vi "gyro-sweeper-V3.vi"() -> ()   [LabVIEW 2018]
uses:
  plot refs -- filter related.ctl
  cursor winow.ctl
  cursor window action.ctl
  KM_file -- read-write control.ctl
  agregator -- action.ctl
  circle corners.ctl
  lorentzian.ctl
  filename-action.ctl
  file -- read-write control.ctl
  publisher action.ctl
  show-win- control.ctl
  data source action.ctl
  cursor action.ctl
  2Dwindow.ctl
  sweper event.ctl
  filename-pattern.ctl
  freq scan type.ctl
  PLL data source.ctl
  peak -- parameters -- complex fit.ctl
  wavepacket.ctl
  filter method control.ctl
  parameters -- scan monitor control.ctl
panel:
  in  "start sweep! :r":bool
  in  "Tab :  Fit":enum32{"complex plane"}(tab)
  in  "fit!":bool=TRUE
  in  "plot staff!":enum16{"plot", "do not plot", "a"}(ring)
  in  "use fast fit!":bool
  out "# of points":dbl=953.475933538175
  out "win center (kHz)":dbl=3399.029286744401
  out "win width (kHz)":dbl=76.27809365793496
  in  "sweeper panel":enum32{"main", "parameters", "save scan"}(tab)
  in  "sweep! :r":bool
  in  "PLL data source":T1=enum."MFLI"
  out "Plot: circle sweep window":cluster{"all rows":dbl[], "all rows":dbl[]}[](graph)
  in  "win":T2={"cen (Hz)"=45005.0594236074, "win (Hz)"=127.23590686512762, "left (Hz)"=44941.44147017484, "right (Hz)"=45068.67737703997}
  in  "history length":i64=5
  out "fit is fine":bool=TRUE
  in  "gamma factor":dbl=1.6
  in  "scan type":T3
  in  "N":i64=250
  in  "Auto-update sweep window!":bool
  out "circle Q":dbl=4152.941585119393 format="%#11_11f"
  out "circle phase (rad)":dbl=0.3233468131446491 format="%#11_11f"
  out "circle gamma (Hz)":dbl=10.835608657224435 format="%#11_11f"
  out "circle frequency (Hz)":dbl=44999.649792667056 format="%#11_11f"
  in  "subtract bgnd!":bool
  in  "save data":enum32{"save/read"}(tab)
  in  "freqsweep name template":T4={"prefix"="RuCl3-rod", "group"="f"}
  in  "Save folder":path=path "/Users/Shared/Data"
  in  "freq sweep file name":string="f020_RuCl3-rod_042518.dat"
  in  "read from disk :l":bool
  in  "read file":path=path "/Users/arkady/Desktop/local_data/TaAs-quirk-Jan2018-losalamos/9w/f006_rucl3_012518.dat"
  in  "Tab :  Fit controls":T5(tab)
  in  "Plot: fragment - filter":cluster{dbl[], dbl[]}[](graph)=[{array[248 elements], array[248 elements]}, {array[248 elements], array[248 elements]}, {array[248 elements], array[248 elements]}, {array[248 elements], array[248 elements]}]
  out "Plot: phase around center":cluster{dbl[], dbl[]}[](graph)
  out "Plot: fragment":cluster{dbl[], dbl[]}[](graph)
  out "Plot: complex plane":cluster{dbl[], dbl[]}[](graph)=[{array[248 elements], array[248 elements]}, {[9.713674760263168e-05, 9.657708189915148e-05, 9.490691105118286e-05, 9.215257465070999e-05, 8.835751022812915e-05, 8.358156821644601e-05, 7.79000680741943e-05, 7.140261045258099e-05, 6.419166413969197e-05, 5.638095006649204e-05, 4.8093647859809984e-05, 3.9460453226039535e-05, 3.061751680177577e-05, 2.1704296976943485e-05, 1.2861360552679704e-05, 4.2281659189092685e-06, -4.059136287772788e-06, -1.186985036097273e-05, -1.9080796673861728e-05, -2.5578254295475043e-05, -3.125975443772674e-05, -3.6035696449409885e-05, -3.983076087199075e-05, -4.258509727246361e-05, -4.4255268120432224e-05, -4.481493382391242e-05, -4.4255268120432224e-05, -4.258509727246361e-05, -3.983076087199072e-05, -3.603569644940987e-05, -3.1259754437726735e-05, -2.5578254295475036e-05, -1.9080796673861714e-05, -1.1869850360972689e-05, -4.059136287772747e-06, 4.2281659189092685e-06, 1.2861360552679719e-05, 2.17042969769435e-05, 3.06175168017758e-05, 3.9460453226039576e-05, 4.809364785980996e-05, 5.638095006649204e-05, 6.419166413969198e-05, 7.1402610452581e-05, 7.790006807419431e-05, 8.358156821644603e-05, 8.835751022812915e-05, 9.215257465071001e-05, 9.490691105118286e-05, 9.657708189915148e-05], [-6.0789908179408565e-05, -5.1894276557869184e-05, -4.3138934360994235e-05, -3.466195856541634e-05, -2.6597036143331644e-05, -1.907135573908757e-05, -1.2203601828282588e-05, -6.102082992687433e-06, -8.630238292101184e-07, 3.430952569479092e-06, 6.712127630475673e-06, 8.928755262988767e-06, 1.0045877925104457e-05, 1.0045877925104457e-05, 8.928755262988753e-06, 6.712127630475673e-06, 3.4309525694790785e-06, -8.630238292101251e-07, -6.102082992687433e-06, -1.2203601828282601e-05, -1.9071355739087562e-05, -2.659703614333165e-05, -3.466195856541635e-05, -4.3138934360994235e-05, -5.18942765578692e-05, -6.0789908179408586e-05, -6.968553980094795e-05, -7.844088199782291e-05, -8.691785779340081e-05, -9.498278021548549e-05, -0.00010250846061972958, -0.00010937621453053454, -0.00011547773336612971, -0.00012071679252960703, -0.00012501076892829625, -0.00012829194398929282, -0.0001305085716218059, -0.0001316256942839216, -0.0001316256942839216, -0.00013050857162180587, -0.00012829194398929282, -0.00012501076892829622, -0.000120716792529607, -0.00011547773336612968, -0.00010937621453053451, -0.00010250846061972952, -9.498278021548549e-05, -8.691785779340079e-05, -7.844088199782288e-05, -6.968553980094791e-05]}, {[3.6089221403832686e-06, 5.864120615280904e-06, 8.11931909017854e-06, 1.0374517565076178e-05, 1.2629716039973813e-05, 1.4884914514871449e-05, 1.7140112989769086e-05, 1.939531146466672e-05, 2.1650509939564358e-05, 2.3905708414461995e-05, 2.616090688935963e-05, 2.8416105364257267e-05, 3.0671303839154904e-05, 3.292650231405254e-05, 3.518170078895017e-05, 3.743689926384781e-05, 3.969209773874545e-05, 4.194729621364308e-05, 4.420249468854072e-05, 4.6457693163438356e-05], [6.507773421354634e-06, -2.219947387216864e-07, -6.951762898798007e-06, -1.3681531058874325e-05, -2.0411299218950647e-05, -2.714106737902697e-05, -3.3870835539103284e-05, -4.0600603699179606e-05, -4.733037185925593e-05, -5.406014001933225e-05, -6.078990817940857e-05, -6.75196763394849e-05, -7.424944449956121e-05, -8.097921265963752e-05, -8.770898081971384e-05, -9.443874897979018e-05, -0.0001011685171398665, -0.00010789828529994281, -0.00011462805346001913, -0.00012135782162009547]}, {[9.345858849012286e-05, 8.672882033004654e-05, 7.999905216997021e-05, 7.32692840098939e-05, 6.653951584981757e-05, 5.980974768974125e-05, 5.307997952966494e-05, 4.6350211369588616e-05, 3.9620443209512294e-05, 3.289067504943597e-05, 2.616090688935965e-05, 1.9431138729283335e-05, 1.270137056920702e-05, 5.971602409130691e-06, -7.581657509456245e-07, -7.487933911021953e-06, -1.4217702071098268e-05, -2.0947470231174584e-05, -2.7677238391250912e-05, -3.440700655132724e-05], [-3.82379234304322e-05, -4.049312190532983e-05, -4.274832038022747e-05, -4.5003518855125107e-05, -4.725871733002275e-05, -4.951391580492038e-05, -5.1769114279818016e-05, -5.402431275471565e-05, -5.627951122961329e-05, -5.853470970451093e-05, -6.0789908179408565e-05, -6.30451066543062e-05, -6.530030512920383e-05, -6.755550360410147e-05, -6.981070207899912e-05, -7.206590055389675e-05, -7.432109902879438e-05, -7.657629750369202e-05, -7.883149597858965e-05, -8.10866944534873e-05]}, {[0.013424540165209643, 0.01681254433898315, 0.02019004611768062, 0.02355493467263274, 0.026905107058024576, 0.030238469525168014, 0.03355293883102678, 0.03684644354017529, 0.04011692531937857, 0.0433623402239834, 0.04658065997531719, 0.049769873228296214, 0.05292798682845071, 0.056053027057581604, 0.0591430408672702, 0.06219609709946967, 0.06521028769341622, 0.0681837288781047, 0.07111456234958441, 0.07400095643233846], [-0.13571760315957762, -0.13533981585140645, -0.1348774553139278, -0.13433081050742715, -0.13370022306711446, -0.13298608708961343, -0.1321888488866639, -0.13130900670619147, -0.13034711042091882, -0.12930376118471318, -0.12817961105688472, -0.1269753625946706, -0.1256917684141598, -0.12432963071993232, -0.12288980080370752, -0.1213731785123146, -0.11978071168531748, -0.11811339556264598, -0.11637227216260333, -0.1145584296306385]}, {[0.01490037751444529, 0.01866106214733388, 0.022410089121688074, 0.02614511541768493, 0.029863806765469864, 0.033563839103999085, 0.037242900033502314, 0.040898690260657164, 0.0445289250355728, 0.048131335579684166, 0.051703670503664666, 0.05524369721447139, 0.05874920331064287, 0.06221799796497817, 0.06564791329373253, 0.06903680571147393, 0.0723825572707546, 0.07568307698575881, 0.07893630213910129, 0.08214019957095828], [-0.15064482340041957, -0.15022547948834955, -0.14971225929174828, -0.14910548355653253, -0.14840553149778546, -0.1476128405627593, -0.14672790615748532, -0.14575128133716095, -0.1446835764605083, -0.14352545880832002, -0.14227765216643043, -0.14094093637337277, -0.13951614683300578, -0.13800417399241327, -0.13640596278540376, -0.13472251204195762, -0.1329548738639908, -0.13110415296782546, -0.1291715059937781, -0.12715814078329715]}, {array[248 elements], array[248 elements]}]
  in  "scale gauge: Plot: complex plane":dbl(slide)=0.00275 min=0.0 max=0.3 step=1e-06 scale=1e-05..0.5 scale format="%#_2g"
  out "lorentzian":T6={"A (VHz)"=0.0007690664340865132, "f (Hz)"=44999.649792667056, "G (Hz)"=10.835608657224435, "phi(rad)"=0.3233468131446491, "Q"=4152.941585119393, "Norm  Ampl"=nan, "bg (V)"=3.608922140383272e-06+6.507773421354641e-06i, "4corners"={"z (-pi/2)"=9.345858849012286e-05-3.8237923430432204e-05i, "z(inf)"=3.608922140383272e-06+6.507773421354641e-06i, "z (pi/2)"=-4.113677471140356e-05-8.334189292838493e-05i, "z center"=2.616090688935963e-05-6.0789908179408565e-05i, "z(0)"=4.871289163833599e-05-0.00012808758978017178i, "radius"=7.097584071327205e-05}} {"bg (V)" format="%#9_9f"; "Q" format="%#9_9f"; "phi(rad)" format="%#9_9f"; "G (Hz)" format="%#9_9f"; "f (Hz)" format="%#9_9f"}
  out "Plot: phase":cluster{"omega out":dbl[], dbl[]}(graph)
  out "Plot: win omega":T8(graph)
  out "Plot: dz/domega":cluster{"omega out":dbl[], dbl[]}(graph)
  in  "Plot: complex plane - filter":cluster{dbl[], dbl[]}[](graph)=[{array[248 elements], array[248 elements]}, {array[248 elements], array[248 elements]}, {[0.0001012150693760883, 0.00010107110703326549, 0.00010063978815839399, 9.992281497002211e-05, 9.892301703377042e-05, 9.764434009532913e-05, 9.609183050840228e-05, 9.427161531905536e-05, 9.219087808506348e-05, 8.985783052569077e-05, 8.728168011378607e-05, 8.447259373809396e-05, 8.144165757918983e-05, 7.820083335738984e-05, 7.476291112530571e-05, 7.114145879135017e-05, 6.73507685734012e-05, 6.340580059394736e-05, 5.932212383931916e-05, 5.511585471601265e-05, 5.080359344659598e-05, 4.6402358556214715e-05, 4.192951970824826e-05, 3.740272915418386e-05, 3.283985206824449e-05, 2.8258896041708113e-05, 2.367794001517175e-05, 1.9115062929232377e-05, 1.458827237516796e-05, 1.0115433527201521e-05, 5.7141986368202625e-06, 1.4019373674035856e-06, -2.8043317559029232e-06, -6.8880085105311325e-06, -1.0832976489984969e-05, -1.4623666707933929e-05, -1.8245119041889463e-05, -2.1683041273973607e-05, -2.4923865495773593e-05, -2.795480165467773e-05, -3.0763888030369817e-05, -3.334003844227453e-05, -3.5673086001647226e-05, -3.775382323563912e-05, -3.9574038424986043e-05, -4.112654801191287e-05, -4.240522495035418e-05, -4.340502288660586e-05, -4.412199607497775e-05, -4.455331494984924e-05, -4.469727729267206e-05, -4.455331494984924e-05, -4.412199607497775e-05, -4.340502288660585e-05, -4.240522495035418e-05, -4.112654801191287e-05, -3.957403842498603e-05, -3.7753823235639105e-05, -3.567308600164721e-05, -3.334003844227452e-05, -3.07638880303698e-05, -2.7954801654677702e-05, -2.4923865495773586e-05, -2.1683041273973594e-05, -1.824511904188945e-05, -1.4623666707933943e-05, -1.0832976489984928e-05, -6.888008510531119e-06, -2.8043317559028826e-06, 1.4019373674035991e-06, 5.7141986368202625e-06, 1.0115433527201551e-05, 1.4588272375167974e-05, 1.9115062929232425e-05, 2.3677940015171765e-05, 2.825889604170811e-05, 3.283985206824452e-05, 3.7402729154183855e-05, 4.1929519708248304e-05, 4.640235855621473e-05, 5.080359344659596e-05, 5.511585471601268e-05, 5.9322123839319156e-05, 6.34058005939474e-05, 6.735076857340121e-05, 7.114145879135022e-05, 7.476291112530574e-05, 7.820083335738984e-05, 8.144165757918985e-05, 8.447259373809397e-05, 8.72816801137861e-05, 8.98578305256908e-05, 9.219087808506348e-05, 9.427161531905536e-05, 9.609183050840228e-05, 9.764434009532913e-05, 9.892301703377042e-05, 9.992281497002211e-05, 0.00010063978815839399, 0.00010107110703326549], [-6.548300655616225e-05, -6.090205052962588e-05, -5.6339173443686514e-05, -5.1812382889622106e-05, -4.7339544041655654e-05, -4.2938309151274406e-05, -3.862604788185772e-05, -3.4419778758551206e-05, -3.0336102003923004e-05, -2.639113402446918e-05, -2.2600443806520194e-05, -1.8978991472564666e-05, -1.5541069240480522e-05, -1.2300245018680544e-05, -9.269308859776414e-06, -6.460222484084306e-06, -3.8840720721795965e-06, -1.5510245128068904e-06, 5.297127211849887e-07, 2.3499279105319138e-06, 3.902437497458743e-06, 5.18111443590005e-06, 6.1809123721517315e-06, 6.897885560523619e-06, 7.32920443539511e-06, 7.4731667782179325e-06, 7.32920443539511e-06, 6.897885560523619e-06, 6.180912372151718e-06, 5.18111443590005e-06, 3.902437497458743e-06, 2.3499279105319002e-06, 5.297127211849751e-07, -1.5510245128069175e-06, -3.88407207217961e-06, -6.460222484084306e-06, -9.269308859776414e-06, -1.230024501868055e-05, -1.5541069240480543e-05, -1.897899147256468e-05, -2.2600443806520187e-05, -2.639113402446918e-05, -3.0336102003923017e-05, -3.441977875855123e-05, -3.862604788185773e-05, -4.293830915127442e-05, -4.7339544041655654e-05, -5.1812382889622106e-05, -5.633917344368653e-05, -6.09020505296259e-05, -6.548300655616228e-05, -7.006396258269862e-05, -7.462683966863799e-05, -7.915363022270241e-05, -8.362646907066887e-05, -8.802770396105013e-05, -9.233996523046681e-05, -9.654623435377329e-05, -0.00010062991110840151, -0.00010457487908785534, -0.00010836556930580432, -0.00011198702163975986, -0.00011542494387184398, -0.00011866576809364396, -0.0001216967042525481, -0.0001245057906282402, -0.00012708194104014492, -0.0001294149885995176, -0.0001314957258335095, -0.00013331594102285643, -0.00013486845060978325, -0.00013614712754822457, -0.00013714692548447624, -0.0001378638986728481, -0.00013829521754771962, -0.00013843917989054242, -0.00013829521754771962, -0.0001378638986728481, -0.0001371469254844762, -0.00013614712754822457, -0.00013486845060978325, -0.0001333159410228564, -0.00013149572583350948, -0.00012941498859951757, -0.0001270819410401449, -0.00012450579062824017, -0.00012169670425254808, -0.00011866576809364396, -0.00011542494387184395, -0.00011198702163975983, -0.00010836556930580426, -0.0001045748790878553, -0.00010062991110840151, -9.654623435377327e-05, -9.233996523046677e-05, -8.802770396105006e-05, -8.362646907066882e-05, -7.91536302227024e-05, -7.462683966863795e-05, -7.006396258269862e-05]}, {[1.899482972370191e-05, 2.042190570156003e-05, 2.536299500300297e-06], [2.1388142418474606e-05, -4.9882036450666976e-05, 1.9102624564056266e-05]}, {[1.6088173004516162e-05, 1.5315829542932655e-05, 1.454348608134915e-05, 1.3771142619765645e-05, 1.299879915818214e-05, 1.2226455696598635e-05, 1.1454112235015128e-05, 1.0681768773431623e-05, 9.909425311848118e-06, 9.13708185026461e-06, 8.364738388681106e-06, 7.5923949270976005e-06, 6.820051465514094e-06, 6.0477080039305886e-06, 5.2753645423470834e-06, 4.503021080763577e-06, 3.7306776191800715e-06, 2.9583341575965664e-06, 2.1859906960130596e-06, 1.4136472344295545e-06], [2.141229803815197e-05, 2.129057954122817e-05, 2.116886104430437e-05, 2.104714254738057e-05, 2.0925424050456767e-05, 2.0803705553532967e-05, 2.0681987056609167e-05, 2.0560268559685368e-05, 2.0438550062761568e-05, 2.0316831565837768e-05, 2.0195113068913965e-05, 2.0073394571990165e-05, 1.9951676075066366e-05, 1.9829957578142566e-05, 1.9708239081218766e-05, 1.9586520584294966e-05, 1.9464802087371166e-05, 1.9343083590447363e-05, 1.9221365093523564e-05, 1.9099646596599764e-05]}, {[2.0421905701560028e-05, 2.1435595251954573e-05, 2.2449284802349118e-05, 2.3462974352743663e-05, 2.447666390313821e-05, 2.5490353453532754e-05, 2.6504043003927302e-05, 2.7517732554321847e-05, 2.8531422104716392e-05, 2.9545111655110937e-05, 3.055880120550548e-05, 3.157249075590003e-05, 3.2586180306294576e-05, 3.359986985668912e-05, 3.4613559407083666e-05, 3.562724895747821e-05, 3.664093850787276e-05, 3.76546280582673e-05, 3.866831760866185e-05, 3.968200715905639e-05], [-4.9882036450666976e-05, -4.9882036450666976e-05, -4.9882036450666976e-05, -4.9882036450666976e-05, -4.9882036450666976e-05, -4.9882036450666976e-05, -4.9882036450666976e-05, -4.9882036450666976e-05, -4.9882036450666976e-05, -4.9882036450666976e-05, -4.9882036450666976e-05, -4.9882036450666976e-05, -4.9882036450666976e-05, -4.9882036450666976e-05, -4.9882036450666976e-05, -4.9882036450666976e-05, -4.9882036450666976e-05, -4.9882036450666976e-05, -4.9882036450666976e-05, -4.9882036450666976e-05]}]
  in  "scale gauge: Plot: complex plane - filter":dbl(slide)=0.000254 min=0.0 max=0.3 step=1e-06 scale=1e-05..0.5 scale format="%#_5g"
  in  "scan monitor control":T9={"gamma acc. frac. - min "=0.3, "gamma acc frac.. - max"=3.0, "peak acc. fraction (af)"=5.0, "min peak acc. window (kHz)"=0.5, "use"=enum."fraction", "abs gamma min(kHz)"=0.005, "abs gamma max(kHz)"=5.0, "# points"=5, "gamma-factor (fa)"=3.0, "interpolate"=enum."line", "init"=TRUE, "Unique strike parameters"=TRUE, "max peak acc. window (kHz)"=10.0, "spacing factor"=1.5, "iterate #"=1, "overwrite ctl?"=FALSE, "write _m files?"=FALSE, "max slope (kHz/sweep)"=0.5, "funnel state"=enum."funnel open"}
  in  "parameters: complex fit":T10={"main VI path"=path "", "scale factor"=3.0, "# of grid points"=200, "parameters: wavepacket"={"R"=0.5, "wave number"=22.0, "delta k"=7.0, "radii vector"=[], "radial section"=[], "wave vector"=22.0, "wavepacket is"=TRUE}, "span"=0.27789, "interference ?"=enum."cp z center", "filter method"=enum."three"} {"span" min=0.0 max=0.5 step=1e-05 scale=0.0001..0.5 scale format="%#_5f"; "parameters: wavepacket"."delta k" format="%#_3f"; "parameters: wavepacket"."wave number" format="%#_3f"; "parameters: wavepacket"."R" format="%#_3f"}
  in  "cursor bracket: fit boundaries":T13={"left"=44877.82351674229, "right "=45005.05942360742, "center"=44941.441470174854, "window"=127.23590686512762, "cursors"=[3, 4, 5], "relative"=0, "absolute"=0, "fixed vertical offset"=0.0, "vertical offset"=0.0, "skew"=0.0, "default window frac"=0.1, "kind"=enum."symmetric", "skew.left"=0.5, "skew.right"=0.5, "Plot ref"=refnum, "wing order"=enum."forw"}
  in  "cursor bracket: circle window":T13={"left"=44941.44147017484, "right "=45068.67737703997, "center"=45005.0594236074, "window"=127.23590686512762, "cursors"=[0, 1, 2], "relative"=0, "absolute"=0, "fixed vertical offset"=0.0, "vertical offset"=0.0, "skew"=0.0, "default window frac"=0.1, "kind"=enum."symmetric", "skew.left"=0.5, "skew.right"=0.5, "Plot ref"=refnum, "wing order"=enum."forw"}
  # "three strikes"
  # "search window"
  # "linear extrapolation"
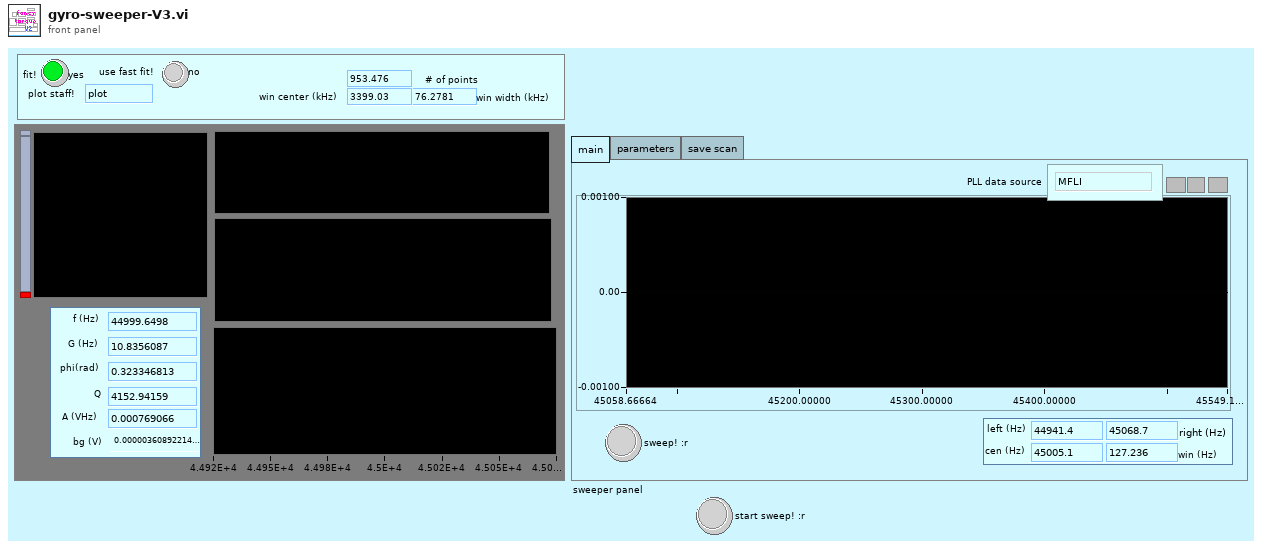
[diagram p1: front panel]
types:
  T1 = typedef "PLL data source.ctl" = enum16{"meta", "MFLI", "SRS865A"}
  T2 = typedef "show-win- control.ctl" = cluster{"cen (Hz)":dbl, "win (Hz)":dbl, "left (Hz)":dbl, "right (Hz)":dbl}
  T3 = typedef "freq scan type.ctl" = enum16{"linear", "arctan"}
  T4 = typedef "filename-pattern.ctl" = cluster{"prefix":string, "group":string}
  T5 = enum32{"complex plane", "complex plane 3", "complex plane 4"}
  T6 = typedef "lorentzian.ctl" = cluster{"A (VHz)":dbl, "f (Hz)":dbl, "G (Hz)":dbl, "phi(rad)":dbl, "Q":dbl, "Norm  Ampl":dbl, "bg (V)":cdb, "4corners":T7}
  T7 = typedef "circle corners.ctl" = cluster{"z (-pi/2)":cdb, "z(inf)":cdb, "z (pi/2)":cdb, "z center":cdb, "z(0)":cdb, "radius":dbl}
  T8 = cluster{"omega out":dbl[], "win omega out":dbl[]}
  T9 = typedef "parameters -- scan monitor control.ctl" = cluster{"gamma acc. frac. - min ":dbl, "gamma acc frac.. - max":dbl, "peak acc. fraction (af)":dbl, "min peak acc. window (kHz)":dbl, "use":enum16{"window", "fraction"}, "abs gamma min(kHz)":dbl, "abs gamma max(kHz)":dbl, "# points":i32, "gamma-factor (fa)":dbl, "interpolate":enum16{"line", "last"}, "init":bool, "Unique strike parameters":bool, "max peak acc. window (kHz)":dbl, "spacing factor":dbl, "iterate #":i32, "overwrite ctl?":bool, "write _m files?":bool, "max slope (kHz/sweep)":dbl, "funnel state":enum16{"funnel open", "funnel closed"}}
  T10 = typedef "peak -- parameters -- complex fit.ctl" = cluster{"main VI path":path, "scale factor":dbl, "# of grid points":i32, "parameters: wavepacket":T11, "span":dbl, "interference ?":enum16{"cp z center", "pm zcenter", "fancy"}, "filter method":T12}
  T11 = typedef "wavepacket.ctl" = cluster{"R":dbl, "wave number":dbl, "delta k":dbl, "radii vector":dbl[], "radial section":cdb[], "wave vector":dbl, "wavepacket is":bool}
  T12 = typedef "filter method control.ctl" = enum16{"four", "five", "one", "two", "three", "zero", "minus one", "minus two"}
  T13 = typedef "cursor winow.ctl" = cluster{"left":dbl, "right ":dbl, "center":dbl, "window":dbl, "cursors":i32[], "relative":i32, "absolute":i32, "fixed vertical offset":dbl, "vertical offset":dbl, "skew":dbl, "default window frac":dbl, "kind":enum16{"symmetric", "skewed", "fancy"}, "skew.left":dbl, "skew.right":dbl, "Plot ref":refnum<vi>, "wing order":enum16{"forw", "back"}}
  T14 = typedef "sweper event.ctl" = enum16{"sweep!", "stop"}
  T15 = typedef "publisher action.ctl" = enum16{"set", "get", "init", "check"}
  T16 = typedef "data source action.ctl" = enum16{"set", "get", "init", "set-and-get"}
  T17 = typedef "cursor window action.ctl" = enum16{"balance", "h. offset change", "cursor moves", "change center", "change window", "init", "check", "reset", "set y to middle", "idle", "-write all Y", "-write left.X", "-write center.X", "-write right.X", "-write all X", "-change center", "-change window", "-change skew", "-read cursor 2", "-read cursor 1", "-read cursor 0", "-read all cursors", "-reset", "-read plot scale", "-set y to middle", "-Q: center.Y is visible", "-Q: window is visible", "-parse center.Y", "-right left from center", "-left move", "-right move", "-set center.Y", "-empty", "-set cursors to default", "-check", "-write center.Y", "-copy cursor 1", "-copy cursor 0", "-copy cursor 2", "move right", "move left", "shrink", "broaden", "skew up", "skew down", "-write plot scale", "zoom X", "change cen&win", "zoom to all data", "color--red", "color--green", "color--yellow", "read", "zoom out", "zoom in", "slide right", "slide left", "set range aspect ratio to 1"}
  T18 = typedef "plot refs -- filter related.ctl" = cluster{"Plot: complex plane - filter":refnum<vi>, "Plot: dz/domega":refnum<vi>, "Plot: fragment filter":refnum<vi>, "Plot: win omega":refnum<vi>, "Plot: phase":refnum<vi>, "Plot: phase around center":refnum<vi>, "Plot: complex plane":refnum<vi>, "Plot: fragment":refnum<vi>}
  T19 = typedef "file -- read-write control.ctl" = enum16{"read", "write all", "append one line"}
  T20 = typedef "filename-action.ctl" = enum16{"rewrite", "parse", "force pattern", "uniquenum"}
  T21 = typedef "KM_file -- read-write control.ctl" = enum16{"read", "write all", "append one line"}
  T22 = typedef "agregator -- action.ctl" = enum16{"append", "interpolate", "empty!", "force", "init", "scale", "read last"}
  T23 = typedef "interpolation state - real.ctl" = cluster{"requested size":i32, "Array":dbl[], "actual number of elements":i32}
  T24 = typedef "2Dwindow.ctl" = cluster{"window y":dbl, "center x":dbl, "center y":dbl, "window x":dbl}
  T25 = typedef "cursor action.ctl" = enum16{"range", "read", "write", "check", "zoom out", "smart zoom out", "zoom to aspect ratio 1", "zoom to win", "zoom out 20%", "zoom in 20%", "-empty", "smart zoom out&aspect", "move range left 20%", "move range right 20%", "move range up 20%", "move range down 20%", "zoom to X win", "zoom to Y win", "zoom out X", "zoom out Y", "zoom in X", "zoom in Y", "check plot scale"}
  T26 = typedef "eventvkey.ctl" = enum16{"ASCII", "Enter", "Return", "Shift", "Ctrl", "Alt", "Cmd", "Opt", "Caps", "NumLock", "Clear", "Break", "Up", "Down", "Left", "Right", "Insert", "Delete", "Home", "End", "PageUp", "PageDown", "Escape", "Help", "Pause", "ScrollLock", "F1", "F2", "F3", "F4", "F5", "F6", "F7", "F8", "F9", "F10", "F11", "F12", "F13", "F14", "F15", "F16", "F17", "F18", "F19", "F20", "F21", "F22", "F23", "F24", "Play", "VolumeUp", "VolumeDown", "Mute", "Two Byte Char"}
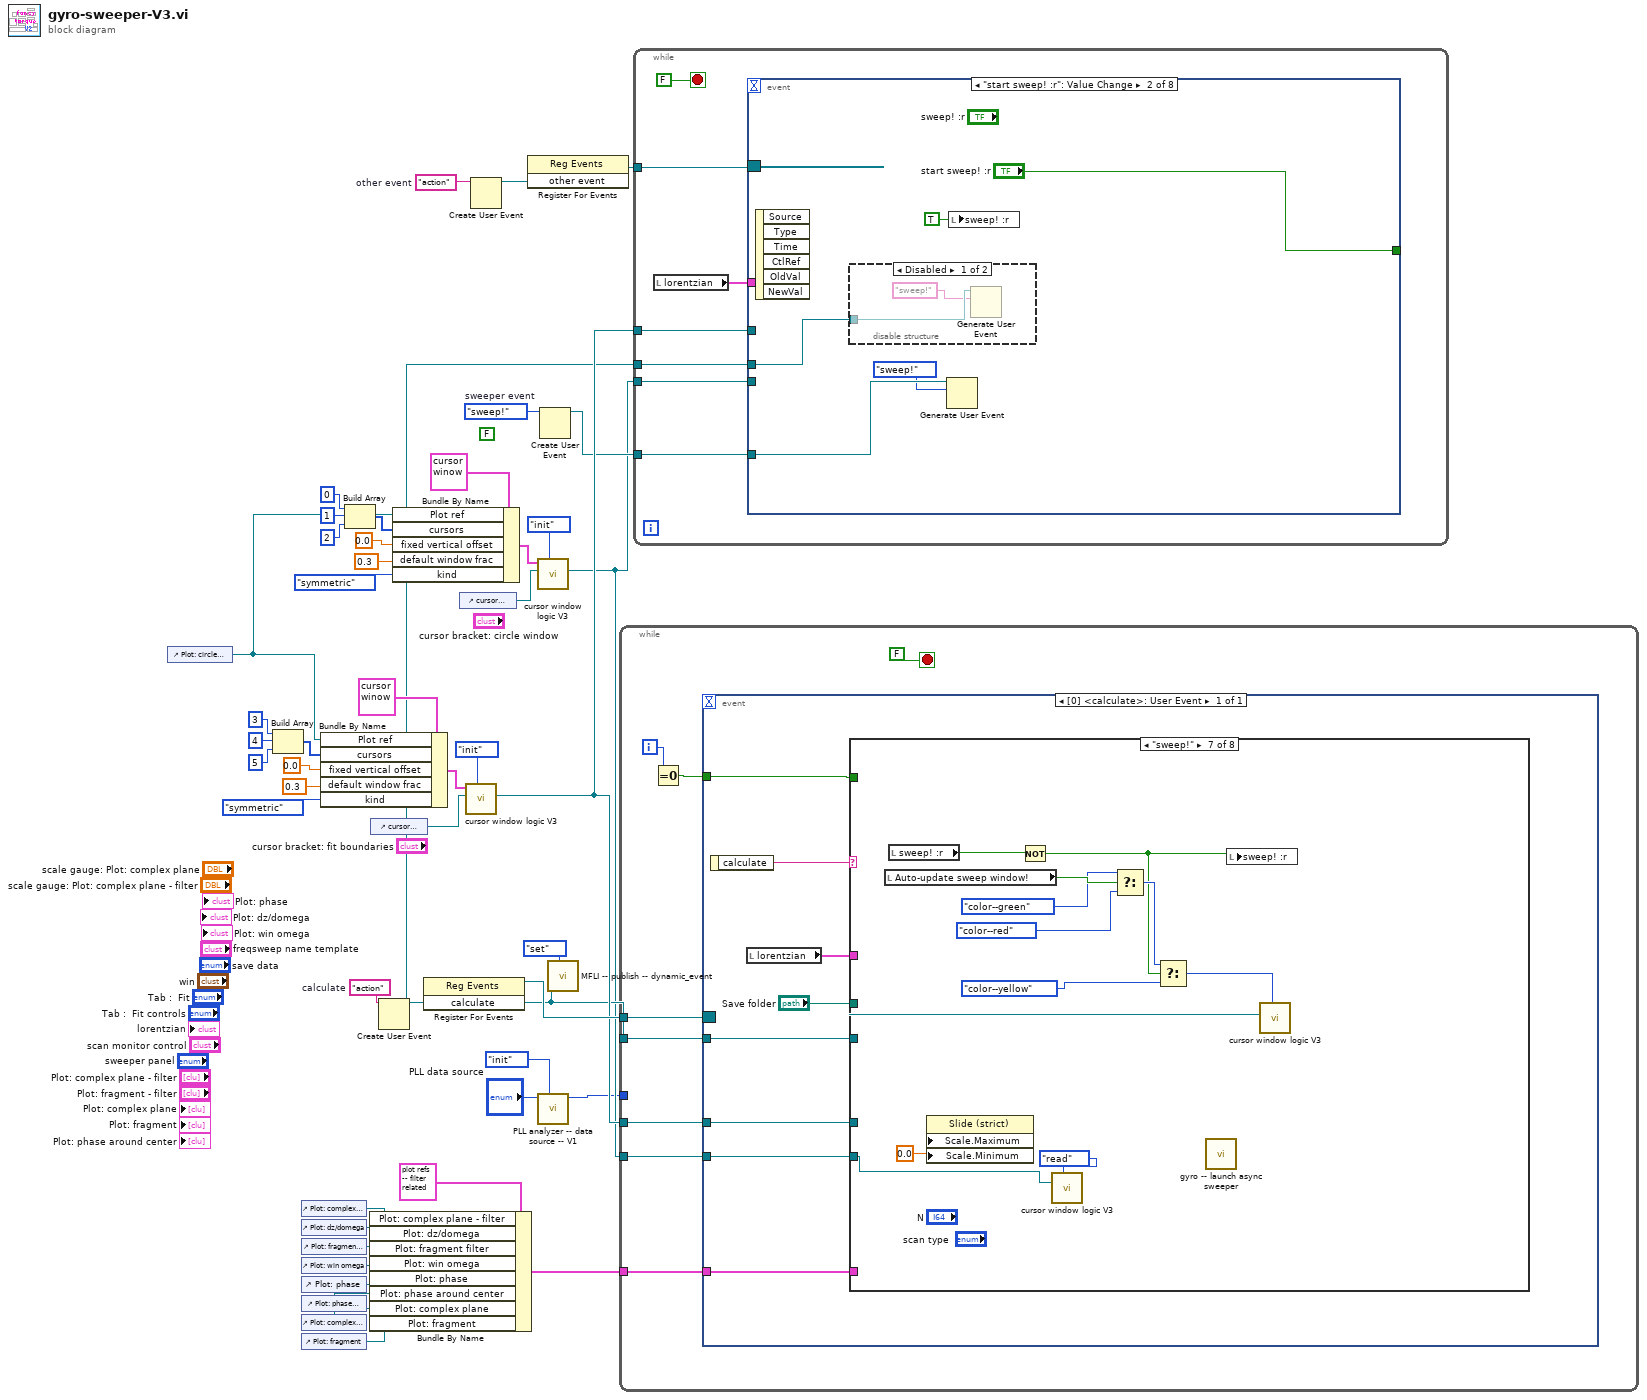
[diagram p0: block diagram]
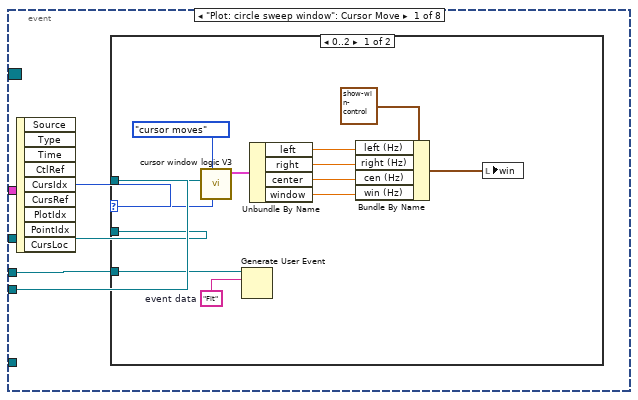
[diagram p2: hidden frame]
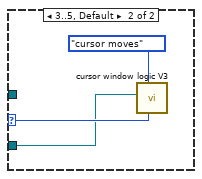
[diagram p3: hidden frame]
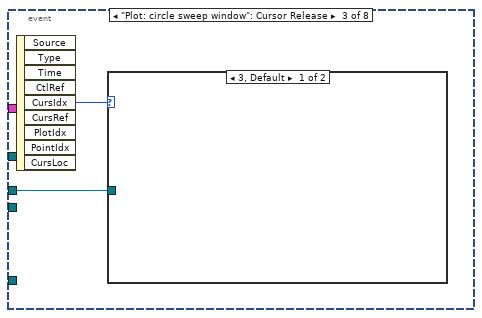
[diagram p5: hidden frame]
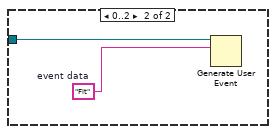
[diagram p6: hidden frame]
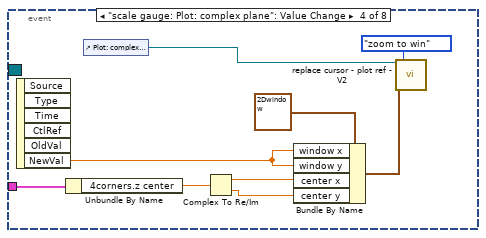
[diagram p7: hidden frame]
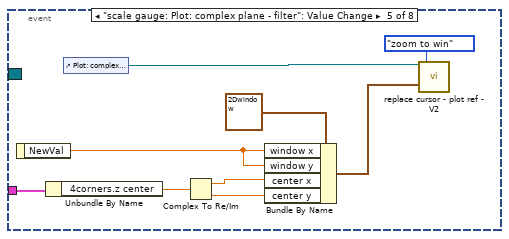
[diagram p8: hidden frame]
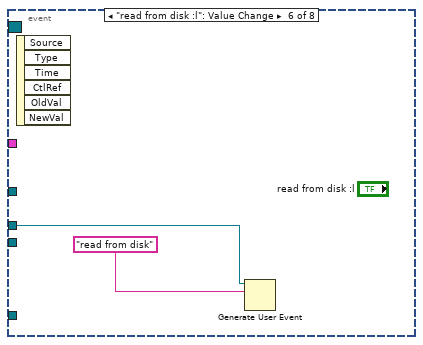
[diagram p9: hidden frame]
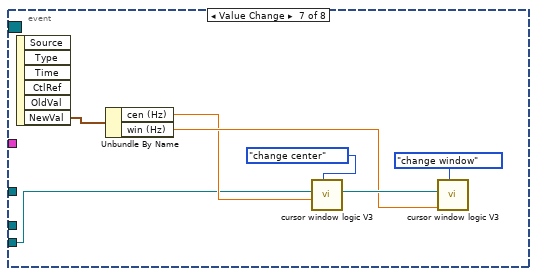
[diagram p10: hidden frame]
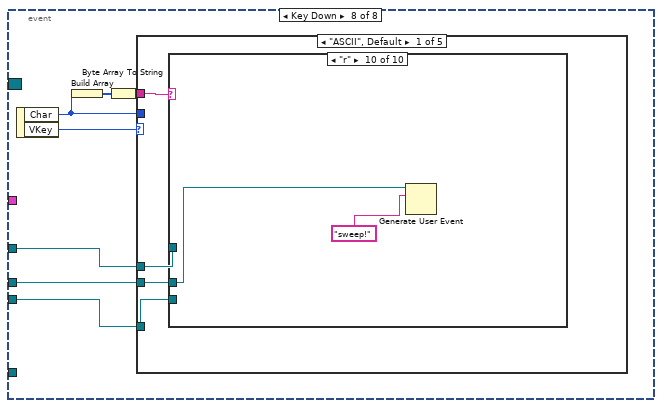
[diagram p11: hidden frame]
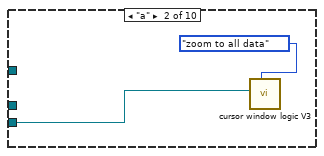
[diagram p13: hidden frame]
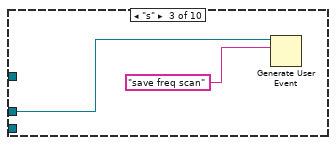
[diagram p14: hidden frame]
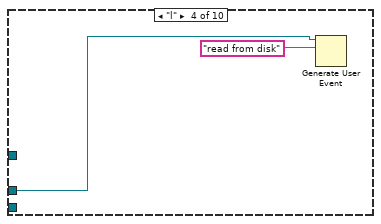
[diagram p15: hidden frame]
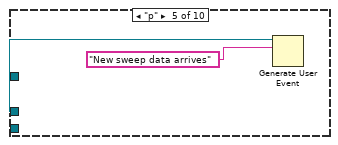
[diagram p16: hidden frame]
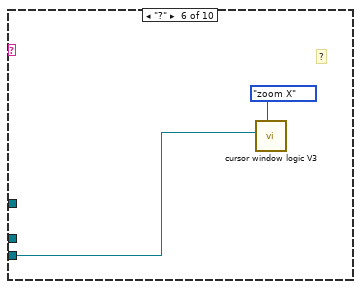
[diagram p17: hidden frame]
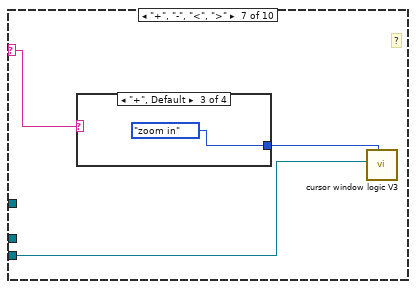
[diagram p18: hidden frame]
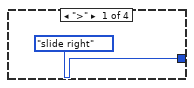
[diagram p19: hidden frame]
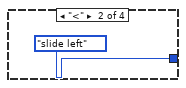
[diagram p20: hidden frame]
diagram:
  w4 = sweper_event."sweep!"  # sweeper event
  w44 = "action"  # other event
  w46 = "action"  # calculate
  (unwired) FALSE
  n1 = control-ref of="Plot: circle sweep window"() -> (w10:refnum<vi>)
  n2 = Build Array(3, 4, 5) -> (w21:i32[])
  n3 = control-ref of="Plot: complex plane - filter"() -> (w41:refnum<vi>)
  n4 = control-ref of="Plot: dz/domega"() -> (w40:refnum<vi>)
  n5 = control-ref of="Plot: fragment - filter"() -> (w39:refnum<vi>)
  n6 = control-ref of="Plot: win omega"() -> (w38:refnum<vi>)
  n7 = control-ref of="Plot: phase"() -> (w37:refnum<vi>)
  n8 = control-ref of="Plot: phase around center"() -> (w35:refnum<vi>)
  n9 = control-ref of="Plot: complex plane"() -> (w34:refnum<vi>)
  n10 = control-ref of="Plot: fragment"() -> (w33:refnum<vi>)
  n11 = Bundle By Name(cluster=T13 {"left"=0.0, "right "=0.0, "center"=0.0, "window"=0.0, "cursors"=[], "relative"=0, "absolute"=0, "fixed vertical offset"=0.0, "vertical offset"=0.0, "skew"=0.0, "default window frac"=0.0, "kind"=enum."symmetric", "skew.left"=0.0, "skew.right"=0.0, "Plot ref"=refnum, "wing order"=enum."forw"} ("cursor bracket: All, data window"), "Plot ref"=w10, "cursors"=w21, "fixed vertical offset"=0.0, "default window frac"=0.3 ("fixed vertical offset"), "kind"=enum16{"symmetric", "skewed", "fancy"}."symmetric") -> (w13:T13)
  n12 = Build Array(0, 1, 2) -> (w32:i32[])
  n13 = Bundle By Name(cluster=T18 {"Plot: complex plane - filter"=refnum, "Plot: dz/domega"=refnum, "Plot: fragment filter"=refnum, "Plot: win omega"=refnum, "Plot: phase"=refnum, "Plot: phase around center"=refnum, "Plot: complex plane"=refnum, "Plot: fragment"=refnum} ("plots: filter related"), "Plot: complex plane - filter"=w41, "Plot: dz/domega"=w40, "Plot: fragment filter"=w39, "Plot: win omega"=w38, "Plot: phase"=w37, "Plot: phase around center"=w35, "Plot: complex plane"=w34, "Plot: fragment"=w33) -> (w36:T18)
  n14 = control-ref of="cursor bracket: fit boundaries"() -> (w11:refnum<vi>)
  n15 = Create User Event(user event datatype=w46) -> (user event=w6:refnum<user-event>)  [unwired: 1 in, 1 out]
  n16 = Bundle By Name(cluster=T13 {"left"=0.0, "right "=0.0, "center"=0.0, "window"=0.0, "cursors"=[], "relative"=0, "absolute"=0, "fixed vertical offset"=0.0, "vertical offset"=0.0, "skew"=0.0, "default window frac"=0.0, "kind"=enum."symmetric", "skew.left"=0.0, "skew.right"=0.0, "Plot ref"=refnum, "wing order"=enum."forw"} ("cursor bracket: All, data window"), "Plot ref"=w10, "cursors"=w32, "fixed vertical offset"=0.0, "default window frac"=0.3 ("fixed vertical offset"), "kind"=enum16{"symmetric", "skewed", "fancy"}."symmetric") -> (w24:T13)
  n17 = register-events(w6) -> (reference out=w47:refnum<event-registration>)  [unwired: 2 in, 1 out]
  n18 = control-ref of="cursor bracket: circle window"() -> (w23:refnum<vi>)
  n19 = call "cursor window logic V3.vi"("cursor window action"=cursor_window_action."init", "cursor window in"=w11, "cursor window init"=w13) -> ("cursor window out"=w9:refnum<vi>)  [unwired: 7 in, 1 out]
  n20 = Create User Event(user event datatype=w44) -> (user event=w43:refnum<user-event>)  [unwired: 1 in, 1 out]
  n21 = register-events(w43) -> (reference out=w45:refnum<event-registration>)  [unwired: 2 in, 1 out]
  n22 = call "cursor window logic V3.vi"("cursor window action"=cursor_window_action."init", "cursor window in"=w23, "cursor window init"=w24) -> ("cursor window out"=w2:refnum<vi>)  [unwired: 7 in, 1 out]
  n23 = call "PLL analyzer -- data source -- V1.vi"("data source action"=data_source_action."init", "PLL data source"="PLL data source") -> ("PLL data source OUT"=w1:T1)  [unwired: 7 in, 2 out]
  n24 = Create User Event(user event datatype=w4) -> (user event=w3:refnum<user-event>)  [unwired: 1 in, 1 out]
  n25 = call "MFLI -- publish -- dynamic_event.vi"("publisher action"=publisher_action."set", "dynamic event"=w6) -> ()  [unwired: 9 in, 1 out]
  n26 = while {
    tunnel: w47 -> [w55]
    tunnel: w6 -> [w53]
    tunnel: w36 -> [w51]
    tunnel: w2 -> [w49]
    tunnel: w9 -> [w48]
    tunnel: w1 -> [_]
    i -> [w52]
    stop <- FALSE stop-if-true
    n27 = Equal To 0?(x=w52) -> (x = 0?=w50:bool)
    n28 = event shown="[0] <calculate>: User Event" {
      selector: w55 -> [_]
      dyn-events: _ -> [_]
      timeout: _ -> [_]
      tunnel: w53 -> [w62]
      tunnel: w51 -> [w60]
      tunnel: w50 -> [w59]
      tunnel: w49 -> [w58]
      tunnel: w48 -> [w56]
      event User Event {
        n29 = event-data() -> ("calculate"=w63:string)  [unwired: 1 in]
        n30 = local read "lorentzian"() -> (w57:T6)
        n31 = case shown="\"sweep!\"" w63 {
          tunnel: w62 -> [w74 w98 w101 _ _ _ _ _]
          tunnel: "Save folder" -> [_ _ _ w125 w147 _ _ _]
          tunnel: w60 -> [_ _ _ _ _ w169 _ _]
          tunnel: w59 -> [_ _ _ _ _ _ _ _]
          tunnel: w58 -> [_ _ _ _ w148 w168 w189 _]
          tunnel: w57 -> [_ _ _ _ w146 _ _ _]
          tunnel: w56 -> [_ _ _ _ w139 _ _ _]
          frame "New sweep data arrives" {
            n32 = call "MFLI -- publish -- freq scan.vi"("publisher action"=publisher_action."get") -> ("Voltage out (V)"=w69:cdb[], "Freq out (Hz)"=w71:dbl[])  [unwired: 9 in]
            n33 = case shown="True" "subtract bgnd!" {
              tunnel: w71 -> [w86 w94]
              tunnel: [w80 w94] -> w70
              tunnel: w69 -> [w82 w93]
              tunnel: [w87 w93] -> w68
              frame True {
                w79 = 10 ("length")
                n34 = Delete From Array(array=w86, length=w79, index=0) -> (array with subset deleted=w85:dbl[])  [unwired: 1 out]
                n35 = Delete From Array(array=w82, length=w79, index=0) -> (array with subset deleted=w81:cdb[])  [unwired: 1 out]
                n36 = call "linear interp iiii- complex - z-omega.vi"("z"=w81, "omega"=w85) -> ("z out"=w88:cdb[], "omega out"=w80:dbl[], "intercept"=w90:cdb, "slope"=w91:cdb)  [unwired: 5 in, 5 out]
                n37 = Multiply(x=w80, y=w91) -> (x*y=w92:cdb[])
                n38 = Add(x=w92, y=w90) -> (x+y=w89:cdb[])
                n39 = Subtract(x=w88, y=w89) -> (x-y=w87:cdb[])
              }
              frame False {
              }
            }
            n40 = Generate User Event(user event=w74, event data cluster="Fit" ("event data")) -> (user event out=w65:refnum<user-event>)  [unwired: 2 in, 1 out]
            n41 = case shown="True" "Auto-update sweep window!" {
              tunnel: w65 -> [_ w95]
              frame False {
              }
              frame True {
                n42 = Generate User Event(user event=w95, event data cluster="Update range" ("event data")) -> ()  [unwired: 2 in, 2 out]
              }
            }
            n43 = Complex To Re/Im(x + iy=w68) -> (x=w77:dbl[], y=w76:dbl[])
            n44 = Bundle("Freq out (Hz)"=w70, w77) -> (w78:cluster{"Freq out (Hz)":dbl[], dbl[]})  [unwired: 1 in]
            n45 = Bundle("Freq out (Hz)"=w70, w76) -> (w75:cluster{"Freq out (Hz)":dbl[], dbl[]})  [unwired: 1 in]
            n46 = Build Array(w78, w75) -> (→"Plot: circle sweep window":cluster{"Freq out (Hz)":dbl[], dbl[]}[])
          }
          frame "sweep off!" {
            n47 = local read "sweep! :r"() -> (w97:bool)
            n48 = case shown="True" w97 {
              tunnel: w98 -> [_ w99]
              frame False {
              }
              frame True {
                n49 = Generate User Event(user event=w99, event data cluster="sweep!" ("event data")) -> ()  [unwired: 2 in, 2 out]
              }
            }
          }
          frame "read from disk" {
            n50 = call "file - read-write - list of lines.vi"("read/write control"=file_--_read-write_control."read", "file path"="read file") -> ("list of lines OUT"=w105:string[])  [unwired: 8 in, 1 out]
            n51 = for {
              tunnel: w105 -> [w115] mode=indexing
              tunnel: [w110] -> w106 mode=indexing
              tunnel: [w109] -> w107 mode=indexing
              w111 = 0.0
              n52 = Scan From String(format string="%f%f%f", input string=w115, default 1=w111, default 2=w111, default 3=w111) -> (output 1=w109:dbl, output 2=w113:dbl, output 3=w112:dbl)  [unwired: 2 in, 3 out]
              n53 = Re/Im To Complex(1:w112, 2:w113) -> (0:w110:cdb)
            }
            n54 = flat-sequence {
              tunnel: w101 -> [w119]
              tunnel: [w119] -> w108
              tunnel: w106 -> [w117]
              tunnel: w107 -> [w116]
              tunnel: w108 -> [w121]
              tunnel: "New sweep data arrives" ("event data") -> [w120]
              frame #0 {
                n55 = call "MFLI -- publish -- freq scan.vi"("publisher action"=publisher_action."set", "Voltage IN (V)"=w117, "Freq IN (Hz)"=w116) -> ()  [unwired: 7 in, 2 out]
              }
              frame #1 {
                n56 = Generate User Event(user event=w121, event data cluster=w120) -> ()  [unwired: 2 in, 2 out]
              }
            }
          }
          frame "save freq scan" {
            n57 = local read "freqsweep name template"() -> (w127:T4)
            n58 = call "MFLI -- publish -- freq scan.vi"("publisher action"=publisher_action."get") -> ("Voltage out (V)"=w122:cdb[], "Freq out (Hz)"=w123:dbl[])  [unwired: 9 in]
            n59 = call "filename-manage.vi"("filename pattern"=w127, "filename-action"=filename-action."uniquenum", "folder"=w125, "file name"="freq sweep file name") -> ("filename OUT"=w126:string)  [unwired: 7 in]
            n60 = call "KM_appendline -- freq sweep.vi"("freq"=w123, "Vout(V)"=w122, "Save frequency scan"=w125, "read/write control"=KM_file_--_read-write_control."append one line", "name or relative path"=w126) -> ()  [unwired: 15 in]
            n61 = local write "freq sweep file name"(w126) -> ()
          }
          frame "Update range" {
            n62 = call "cursor window logic V3.vi"("cursor window action"=cursor_window_action."read", "cursor window in"=w139) -> ("cursor window out"=w142:T13)  [unwired: 8 in, 1 out]
            n63 = Unbundle By Name(w142) -> ("left"=w141:dbl, "right"=w140:dbl, "window"=w134:dbl)
            n64 = Unbundle By Name(w146) -> ("f (Hz)"=w137:dbl, "G (Hz)"=w144:dbl)
            n65 = Multiply(x=w134, y=3.0 ("lower")) -> (x*y=w135:dbl)
            n66 = Multiply(x=w134, y=0.0003 ("lower")) -> (x*y=w132:dbl)
            n67 = call "Q -- check range -- i -- real.vi"("upper"=w140, "lower"=w141, "number"=w137) -> ("in range?"=w145:bool)  [unwired: 6 in, 2 out]
            n68 = call "Q -- check range -- i -- real.vi"("upper"=w135, "lower"=w132, "number"=w144) -> ("in range?"=w143:bool)  [unwired: 6 in, 2 out]
            n69 = And(x=w145, y=w143) -> (x .and. y?=w138:bool)
            "fit is fine" <- w138
            n70 = case shown="True" w138 {
              tunnel: w144 -> [_ w156]
              tunnel: w137 -> [_ w151]
              tunnel: w148 -> [_ w157]
              tunnel: w147 -> [_ _]
              frame False {
              }
              frame True {
                (unwired) agregator_--_action."append" ("aggregator action")
                n71 = for {
                  N: 1 -> [_]
                  tunnel: "history length" -> [w161]
                  tunnel: w151 -> [w166]
                  shift-right: [w162] -> _
                  shift-left: _ -> [w165]
                  tunnel: [w159] -> w150
                  n72 = call "aggregator - vii - real - atomic.vi"("aggregator action"=agregator_--_action."append", "requested size"=w161, "number"=w166, "state IN"=w165) -> ("state OUT"=w163:T23)  [unwired: 4 in, 3 out]
                  n73 = call "aggregator - vii - real - atomic.vi"("aggregator action"=agregator_--_action."interpolate", "requested size"=w161, "state IN"=w163) -> ("interp average"=w159:dbl, "state OUT"=w162:T23)  [unwired: 5 in, 2 out]
                }
                n74 = Compound Arithmetic op=MULTIPLY("gamma factor", w156, 2.0 ("value")) -> (w154:dbl)
                n75 = call "cursor window logic V3.vi"("cursor window action"=cursor_window_action."change cen&win", "window"=w154, "center"=w150, "cursor window in"=w157) -> ()  [unwired: 6 in, 2 out]
              }
            }
          }
          frame "Fit" {
            n76 = case shown="True" "fit!" {
              tunnel: w169 -> [_ w184]
              tunnel: w168 -> [_ w182]
              frame False {
                (unwired) T6 {"A (VHz)"=-1.0311345636926572, "f (Hz)"=-1.0311345636926572, "G (Hz)"=-1.0311345636926572, "phi(rad)"=-1.0311345636926572, "Q"=-1.0311345636926572, "Norm  Ampl"=-1.0311345636926572, "bg (V)"=-1.0311345636926572+0.0i, "4corners"={"z (-pi/2)"=-1.0311345636926572+0.5736824521422934i, "z(inf)"=-0.5200164984937075+1.0975277942502903i, "z (pi/2)"=-1.0311345636926572+0.5736824521422934i, "z center"=-0.5136528600391839+0.580046090596817i, "z(0)"=-0.5200164984937075+1.0975277942502903i, "radius"=-1.0311345636926572}} ("pm lorentzian")
              }
              frame True {
                n77 = call "MFLI -- publish -- freq scan.vi"("publisher action"=publisher_action."get") -> ("Voltage out (V)"=w170:cdb[], "Freq out (Hz)"=w171:dbl[])  [unwired: 9 in]
                n78 = call "cursor window logic V3.vi"("cursor window action"=cursor_window_action."read", "cursor window in"=w182) -> ("cursor window out"=w179:T13)  [unwired: 8 in, 1 out]
                n79 = call "acquire cursor window data.vi"("z in"=w170, "omega in"=w171, "cursor window"=w179) -> ("z out"=w180:cdb[], "omega  out"=w181:dbl[])  [unwired: 4 in, 3 out]
                n80 = call "KM_peak -- find -- pm - V1.vi"("omega in"=w181, "z in"=w180, "parameters: complex fit"="parameters: complex fit", "plots: filter related"=w184, "plot staff ?"="plot staff!", "just guess?"="use fast fit!", "subtract linear BG"=FALSE) -> ("pm lorentzian"=w173:T6)  [unwired: 10 in, 2 out]
                n81 = Unbundle By Name(w173) -> ("f (Hz)"=→"circle frequency (Hz)":dbl, "G (Hz)"=→"circle gamma (Hz)":dbl, "phi(rad)"=→"circle phase (rad)":dbl, "Q"=→"circle Q":dbl)
                n82 = local write "lorentzian"(w173) -> ()
                n83 = call "publish -- lorentzian.vi"("publisher action"=publisher_action."set", "lorentzian IN"=w173) -> ()  [unwired: 9 in, 1 out]
              }
            }
          }
          frame "sweep!" {
            n84 = local read "Auto-update sweep window!"() -> (w198:bool)
            n85 = local read "sweep! :r"() -> (w197:bool)
            n86 = property class="Slide (strict)" props=["Scale", "Maximum", "Scale", "Minimum"]("Scale.Minimum"=0.0 ("Data Entry Limits:Minimum")) -> ()  [unwired: 3 in, 2 out]
            n87 = Not(x=w197) -> (.not. x?=w195:bool)
            n88 = call "cursor window logic V3.vi"("cursor window action"=cursor_window_action."read", "cursor window in"=w189) -> ()  [unwired: 8 in, 2 out]
            n89 = Select(t=cursor_window_action."color--green" ("cursor window action"), s=w198, f=cursor_window_action."color--red" ("cursor window action")) -> (s? t:f=w199:T17)
            n90 = Select(t=w199, s=w195, f=cursor_window_action."color--yellow" ("cursor window action")) -> (s? t:f=w196:T17)
            n91 = call "gyro -- launch async sweeper.vi"() -> ()  [unwired: 11 in, 1 out]
            n92 = local write "sweep! :r"(w195) -> ()
            n93 = call "cursor window logic V3.vi"("cursor window action"=w196, "cursor window in"=w189) -> ()  [unwired: 8 in, 2 out]
          }
          frame "Void", Default {
          }
        }
      }
    }
  }
  n94 = while {
    tunnel: w45 -> [w206]
    tunnel: w6 -> [w205]
    tunnel: w2 -> [w204]
    tunnel: w9 -> [w201]
    tunnel: w3 -> [w200]
    stop <- FALSE stop-if-true
    n95 = local read "lorentzian"() -> (w203:T6)
    n96 = event shown="[1] \"start sweep! :r\": Value Change" {
      selector: w206 -> [_ _ _ _ _ _ _ _]
      dyn-events: _ -> [_ _ _ _ _ _ _ _]
      timeout: _ -> [_ _ _ _ _ _ _ _]
      tunnel: w205 -> [w207 w229 w234 _ _ w256 _ w269]
      tunnel: w204 -> [w210 _ _ _ _ _ w257 w265]
      tunnel: w203 -> [_ _ _ w244 w253 _ _ _]
      tunnel: w201 -> [w208 _ _ _ _ _ _ w264]
      tunnel: [_ "start sweep! :r" _ _ _ _ _ _] -> _
      tunnel: w200 -> [_ w228 _ _ _ _ _ _]
      event "Plot: circle sweep window": Cursor Move {
        n97 = event-data() -> ("CursIdx"=w209:i32)  [unwired: 1 in, 8 out]
        n98 = case shown="0..2" w209 {
          selector: w209 -> [w220 w224]
          tunnel: w210 -> [w222 _]
          tunnel: w208 -> [_ w223]
          tunnel: w207 -> [w218 _]
          frame 0..2 {
            w217 = "Fit"  # event data
            n99 = call "cursor window logic V3.vi"("CursIdx"=w220, "cursor window action"=cursor_window_action."cursor moves", "cursor window in"=w222) -> ("cursor window out"=w219:T13)  [unwired: 7 in, 1 out]
            n100 = Generate User Event(user event=w218, event data cluster=w217) -> ()  [unwired: 2 in, 2 out]
            n101 = Unbundle By Name(w219) -> ("left"=w214:dbl, "right"=w213:dbl, "center"=w212:dbl, "window"=w211:dbl)
            n102 = Bundle By Name(cluster=T2 {"cen (Hz)"=-0.35260838541595674, "win (Hz)"=17.234446484426172, "left (Hz)"=-8.969831627629043, "right (Hz)"=8.26461485679713} ("win"), "left (Hz)"=w214, "right (Hz)"=w213, "cen (Hz)"=w212, "win (Hz)"=w211) -> (w215:T2)
            n103 = local write "win"(w215) -> ()
          }
          frame 3..5, Default {
            n104 = call "cursor window logic V3.vi"("CursIdx"=w224, "cursor window action"=cursor_window_action."cursor moves", "cursor window in"=w223) -> ()  [unwired: 7 in, 2 out]
          }
        }
      }
      event "start sweep! :r": Value Change {
        n105 = event-data() -> ()  [unwired: 1 in, 6 out]
        n106 = disable-structure shown="Disabled" {
          disable-tunnel: w229 -> [w232 _]
          frame Disabled {
            n107 = Generate User Event(user event=w232, event data cluster="sweep!" ("event data")) -> ()  [unwired: 2 in, 2 out]
          }
          frame Enabled {
          }
        }
        n108 = Generate User Event(user event=w228, event data cluster=sweper_event."sweep!" ("event data")) -> ()  [unwired: 2 in, 2 out]
        n109 = local write "sweep! :r"(TRUE ("sweep! :r")) -> ()
      }
      event "Plot: circle sweep window": Cursor Release {
        n110 = event-data() -> ("CursIdx"=w233:i32)  [unwired: 1 in, 8 out]
        n111 = case shown="3, Default" w233 {
          tunnel: w234 -> [_ w235]
          frame 3, Default {
          }
          frame 0..2 {
            w236 = "Fit"  # event data
            n112 = Generate User Event(user event=w235, event data cluster=w236) -> ()  [unwired: 2 in, 2 out]
          }
        }
      }
      event "scale gauge: Plot: complex plane": Value Change {
        n113 = event-data() -> ("NewVal"=w238:dbl)  [unwired: 1 in, 5 out]
        n114 = Unbundle By Name(w244) -> ("4corners.z center"=w245:cdb)
        n115 = control-ref of="Plot: complex plane"() -> (w243:refnum<vi>)
        n116 = Complex To Re/Im(x + iy=w245) -> (x=w240:dbl, y=w239:dbl)
        n117 = Bundle By Name(cluster=T24 {"window y"=0.0021014740628288917, "center x"=44850.89441339177, "center y"=2.5658109925320947, "window x"=17480.201988350764} ("window IN"), "window x"=w238, "window y"=w238, "center x"=w240, "center y"=w239) -> (w237:T24)
        n118 = call "replace cursor - plot ref - V2.vi"("Plot ref in"=w243, "window IN"=w237, "cursor action"=cursor_action."zoom to win") -> ()  [unwired: 13 in, 4 out]
      }
      event "scale gauge: Plot: complex plane - filter": Value Change {
        n119 = event-data() -> ("NewVal"=w248:dbl)  [unwired: 1 in]
        n120 = Unbundle By Name(w253) -> ("4corners.z center"=w254:cdb)
        n121 = control-ref of="Plot: complex plane - filter"() -> (w249:refnum<vi>)
        n122 = Complex To Re/Im(x + iy=w254) -> (x=w247:dbl, y=w246:dbl)
        n123 = Bundle By Name(cluster=T24 {"window y"=0.0021014740628288917, "center x"=44850.89441339177, "center y"=2.5658109925320947, "window x"=17480.201988350764} ("window IN"), "window x"=w248, "window y"=w248, "center x"=w247, "center y"=w246) -> (w250:T24)
        n124 = call "replace cursor - plot ref - V2.vi"("Plot ref in"=w249, "window IN"=w250, "cursor action"=cursor_action."zoom to win") -> ()  [unwired: 13 in, 4 out]
      }
      event "read from disk :l": Value Change {
        n125 = event-data() -> ()  [unwired: 1 in, 6 out]
        n126 = Generate User Event(user event=w256, event data cluster="read from disk" ("event data")) -> ()  [unwired: 2 in, 2 out]
      }
      event Value Change {
        n127 = event-data() -> ("NewVal"=w260:T2)  [unwired: 1 in, 5 out]
        n128 = Unbundle By Name(w260) -> ("cen (Hz)"=w258:dbl, "win (Hz)"=w259:dbl)
        n129 = call "cursor window logic V3.vi"("cursor window action"=cursor_window_action."change center", "center"=w258, "cursor window in"=w257) -> ("cursor window out"=w261:refnum<vi>)  [unwired: 7 in, 1 out]
        n130 = call "cursor window logic V3.vi"("cursor window action"=cursor_window_action."change window", "window"=w259, "cursor window in"=w261) -> ()  [unwired: 7 in, 2 out]
      }
      event Key Down {
        n131 = event-data() -> ("Char"=w267:i16, "VKey"=w270:T26)  [unwired: 1 in]
        n132 = Build Array(w267) -> (w268:i16[])
        n133 = Byte Array To String(unsigned byte array=w268) -> (string=w266:string)
        n134 = case shown="\"ASCII\", Default" w270 {
          selector: w270 -> [_ _ _ _ w315]
          tunnel: w267 -> [_ _ _ _ _]
          tunnel: w269 -> [w274 _ _ _ w314]
          tunnel: w266 -> [w273 _ _ _ _]
          tunnel: w265 -> [w271 _ _ _ w311]
          tunnel: w264 -> [w272 _ _ _ _]
          frame "ASCII", Default {
            n135 = case shown="\"r\"" w273 {
              selector: w273 -> [_ _ _ _ _ _ w286 _ _ _]
              tunnel: w274 -> [_ _ w277 w279 w281 _ _ _ _ w302]
              tunnel: w271 -> [_ w275 _ _ _ w283 w287 w294 w301 _]
              tunnel: w272 -> [_ _ _ _ _ _ _ w292 _ _]
              frame "0", Default {
              }
              frame "a" {
                n136 = call "cursor window logic V3.vi"("cursor window action"=cursor_window_action."zoom to all data", "cursor window in"=w275) -> ()  [unwired: 8 in, 2 out]
              }
              frame "s" {
                n137 = Generate User Event(user event=w277, event data cluster="save freq scan" ("event data")) -> ()  [unwired: 2 in, 2 out]
              }
              frame "l" {
                n138 = Generate User Event(user event=w279, event data cluster="read from disk" ("event data")) -> ()  [unwired: 2 in, 2 out]
              }
              frame "p" {
                n139 = Generate User Event(user event=w281, event data cluster="New sweep data arrives" ("event data")) -> ()  [unwired: 2 in, 2 out]
              }
              frame "?" {
                # "?"
                n140 = call "cursor window logic V3.vi"("cursor window action"=cursor_window_action."zoom X", "cursor window in"=w283) -> ()  [unwired: 8 in, 2 out]
              }
              frame "+", "-", "<", ">" {
                # "?"
                n141 = case shown="\"+\", Default" w286 {
                  tunnel: [cursor_window_action."slide right" ("cursor window action") cursor_window_action."slide left" ("cursor window action") cursor_window_action."zoom in" ("cursor window action") cursor_window_action."zoom out" ("cursor window action")] -> w285
                  frame ">" {
                  }
                  frame "<" {
                  }
                  frame "+", Default {
                  }
                  frame "-" {
                  }
                }
                n142 = call "cursor window logic V3.vi"("cursor window action"=w285, "cursor window in"=w287) -> ()  [unwired: 8 in, 2 out]
              }
              frame "c" {
                n143 = call "cursor window logic V3.vi"("cursor window action"=cursor_window_action."check", "cursor window in"=w292) -> ()  [unwired: 8 in, 2 out]
                n144 = call "cursor window logic V3.vi"("cursor window action"=cursor_window_action."check", "cursor window in"=w294) -> ()  [unwired: 8 in, 2 out]
              }
              frame "t" {
                n145 = local read "Auto-update sweep window!"() -> (w300:bool)
                n146 = Not(x=w300) -> (.not. x?=w299:bool)
                n147 = local write "Auto-update sweep window!"(w299) -> ()
                n148 = Select(t=cursor_window_action."color--green" ("cursor window action"), s=w299, f=cursor_window_action."color--red" ("cursor window action")) -> (s? t:f=w296:T17)
                n149 = call "cursor window logic V3.vi"("cursor window action"=w296, "cursor window in"=w301) -> ()  [unwired: 8 in, 2 out]
              }
              frame "r" {
                n150 = Generate User Event(user event=w302, event data cluster="sweep!" ("event data")) -> ()  [unwired: 2 in, 2 out]
              }
            }
          }
          frame "Escape" {
          }
          frame "PageUp" {
          }
          frame "PageDown" {
          }
          frame "Up".."Right" {
            w304 = "Fit"  # event data
            n151 = case shown="\"Left\"" w315 {
              tunnel: [cursor_window_action."move right" ("cursor window action") cursor_window_action."move left" ("cursor window action") cursor_window_action."broaden" ("cursor window action") cursor_window_action."shrink" ("cursor window action")] -> w313
              frame "Right", Default {
              }
              frame "Left" {
              }
              frame "Up" {
              }
              frame "Down" {
              }
            }
            n152 = call "cursor window logic V3.vi"("cursor window action"=w313, "cursor window in"=w311) -> ("cursor window out"=w312:T13)  [unwired: 8 in, 1 out]
            n153 = Unbundle By Name(w312) -> ("left"=w308:dbl, "right"=w307:dbl, "center"=w306:dbl, "window"=w305:dbl)
            n154 = Generate User Event(user event=w314, event data cluster=w304) -> ()  [unwired: 2 in, 2 out]
            n155 = Bundle By Name(cluster=T2 {"cen (Hz)"=-0.35260838541595674, "win (Hz)"=17.234446484426172, "left (Hz)"=-8.969831627629043, "right (Hz)"=8.26461485679713} ("win"), "left (Hz)"=w308, "right (Hz)"=w307, "cen (Hz)"=w306, "win (Hz)"=w305) -> (w310:T2)
            n156 = local write "win"(w310) -> ()
          }
        }
      }
    }
  }
